vi "INST_PS_SET_VOLTAGE_LEVEL_2.0.0.vi"(4 "Use OPC(T)":bool, 6 "Instrument Select (Output 1)":string(combo), 8 "error in (no error)":errorcluster, 9 "Voltage (0.0)":dbl format="%.2p", 10 "Voltage (0.0)str":string, 11 "VISA session":refnum<visa-resource-name>) -> (0 "error out":errorcluster, 3 "dup VISA session":refnum<visa-resource-name>)   [LabVIEW 2018]
doc: "This VI configures the DC voltage level the power supply attempts to generate."
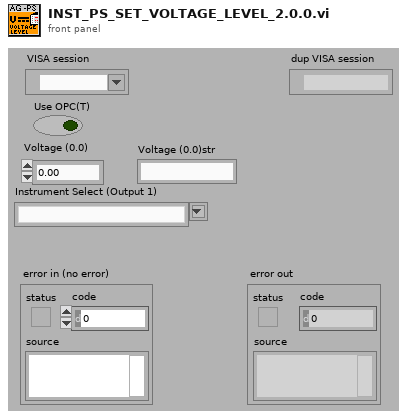
[diagram p1: front panel]
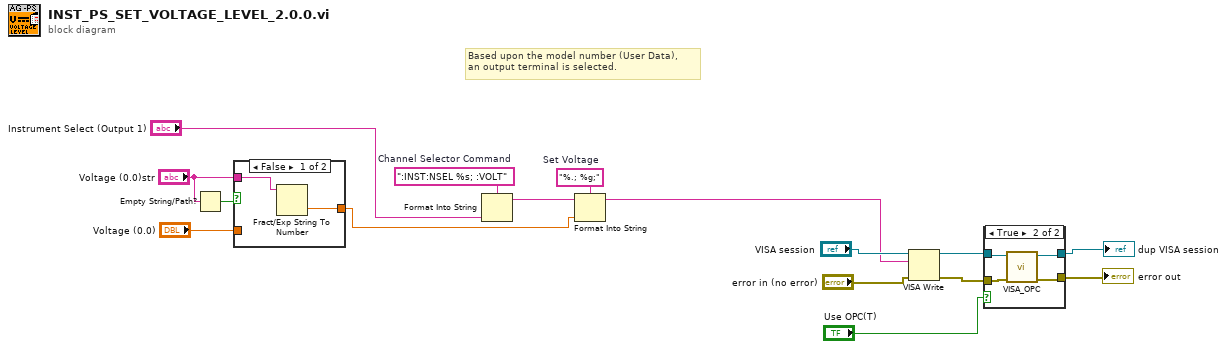
[diagram p0: block diagram]
diagram:
  w14 = ":INST:NSEL %s; :VOLT"  # Channel Selector Command
  w16 = "%.; %g;"  # Set Voltage
  # "Based upon the model number (User Data), \nan output terminal is selected."
  n1 = Empty String/Path?(string/path="Voltage (0.0)str") -> (empty?=w4:bool)
  n2 = case shown="False" w4 {
    tunnel: "Voltage (0.0)str" -> [w18 _]
    tunnel: [w17 w19] -> w3
    tunnel: "Voltage (0.0)" -> [_ w19]
    frame False {
      n3 = Fract/Exp String To Number(string=w18) -> (number=w17:dbl)  [unwired: 3 in, 1 out]
    }
    frame True {
    }
  }
  n4 = Format Into String(format string=w14, "Instrument Select (Output 1)") -> (resulting string=w15:string)  [unwired: 2 in, 1 out]
  n5 = Format Into String(format string=w16, initial string=w15, w3) -> (resulting string=w1:string)  [unwired: 1 in, 1 out]
  n6 = VISA Write(VISA resource name="VISA session", write buffer=w1, error in (no error)="error in (no error)") -> (VISA resource name out=w13:refnum<visa-resource-name>, error out=w12:errorcluster)  [unwired: 1 out]
  n7 = case shown="True" "Use OPC(T)" {
    tunnel: w12 -> [w21 w24]
    tunnel: [w21 w25] -> w9
    tunnel: w13 -> [w20 w23]
    tunnel: [w20 w22] -> w10
    frame False {
    }
    frame True {
      n8 = call "VISA_OPC.vi"("error in"=w24, "Session In"=w23) -> ("error out"=w25:errorcluster, "Session Out"=w22:refnum<visa-resource-name>)  [unwired: 7 in, 1 out]
    }
  }
  "error out" <- w9
  "dup VISA session" <- w10
